vi "Initialize.vi"(8 "error in (no error)":errorcluster, 11 "Bronkhorst Settings in":T1) -> (0 "error out":errorcluster, 2 "No Meter Connected":bool, 3 "Bronkhorst Settings out":T1)   [LabVIEW 2018, in "Bronkhorst M14 Flow Meter.lvlib"]
uses:
  Bronkhorst M14 Flow Meter.lvlib
  Settings Cluster.ctl
  <vilib>/Instr/_visa.llb/VISA Configure Serial Port (Instr).vi
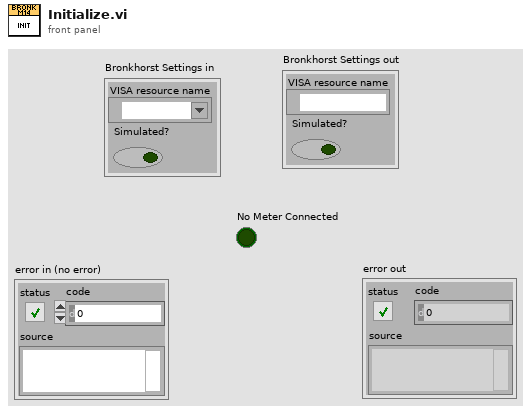
[diagram p1: front panel]
types:
  T1 = typedef "Bronkhorst M14 Flow Meter.lvlib/Settings Cluster.ctl" = cluster{"VISA resource name":refnum<visa-resource-name>, "Simulated?":bool}
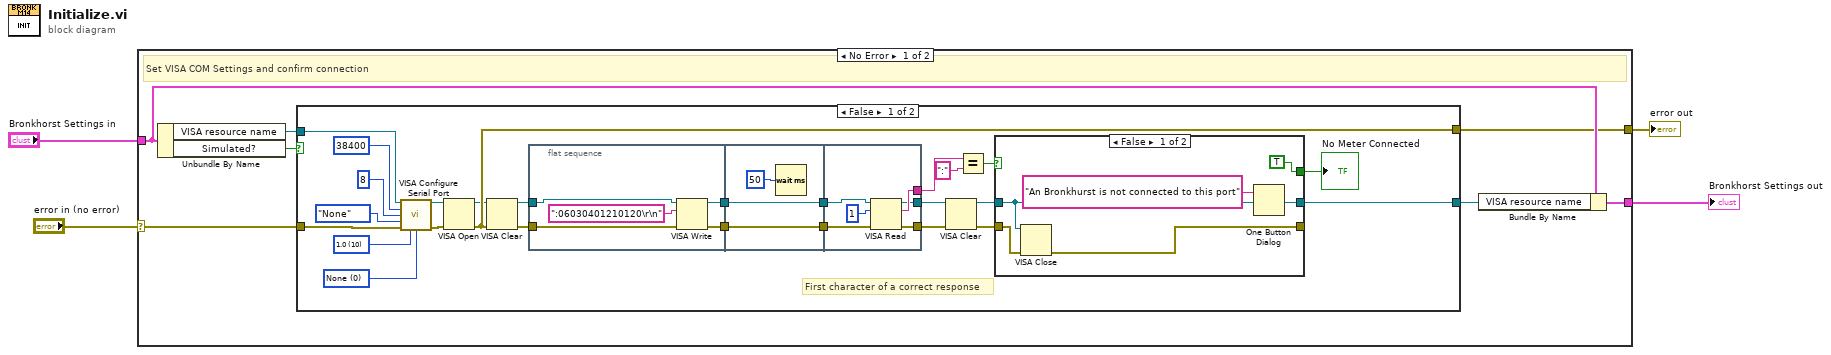
[diagram p0: block diagram]
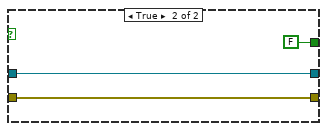
[diagram p2: hidden frame]
diagram:
  n1 = case shown="No Error" "error in (no error)" {
    selector: "error in (no error)" -> [w11 w63]
    tunnel: "Bronkhorst Settings in" -> [w9 w62]
    tunnel: [w5 w63] -> w3
    tunnel: [w8 w62] -> w1
    frame No Error {
      # "Set VISA COM Settings and confirm connection"
      n2 = Unbundle By Name(w9) -> ("VISA resource name"=w7:refnum<visa-resource-name>, "Simulated?"=w10:bool)
      n3 = case shown="False" w10 {
        tunnel: w11 -> [w31 w61]
        tunnel: [w28 w61] -> w5
        tunnel: w7 -> [w29 w60]
        tunnel: [w16 w60] -> w6
        frame False {
          w33 = u16 0 items=["None", "XON/XOFF", "RTS/CTS", "XON/XOFF & RTS/CTS", "DTR/DSR", "XON/XOFF & DTR/DSR"] ("flow control (0:none)")
          w34 = u16 10 items=["1.0"=10, "1.5"=15, "2.0"=20] ("stop bits (10: 1 bit)")
          # "First character of a correct response"
          n4 = call-poly "VISA Configure Serial Port"("VISA resource name"=w29, "baud rate (9600)"=u32 38400, "data bits (8)"=u16 8, "parity (0:none)"=enum16{"None", "Odd", "Even", "Mark", "Space"}."None", "error in (no error)"=w31, "stop bits (10: 1 bit)"=w34, "flow control (0:none)"=w33) -> ("VISA resource name out"=w30:refnum<visa-resource-name>, "error out"=w32:errorcluster)  [unwired: 7 in]
          n5 = VISA Open(error in (no error)=w32, VISA resource name=w30) -> (VISA resource name=w13:refnum<visa-resource-name>, error out=w28:errorcluster)  [unwired: 3 in]
          n6 = VISA Clear(VISA resource name=w13, error in (no error)=w28) -> (VISA resource name out=w14:refnum<visa-resource-name>, error out=w15:errorcluster)
          n7 = flat-sequence {
            tunnel: w15 -> [w42]
            tunnel: [w40] -> w27
            tunnel: [w39] -> w26
            tunnel: w14 -> [w38]
            tunnel: w27 -> [w45]
            tunnel: [w45] -> w25
            tunnel: w26 -> [w44]
            tunnel: [w44] -> w24
            tunnel: [w51] -> w18
            tunnel: [w50] -> w22
            tunnel: [w49] -> w17
            tunnel: w25 -> [w48]
            tunnel: w24 -> [w47]
            frame #0 {
              n8 = VISA Write(VISA resource name=w38, write buffer=":06030401210120\r\n", error in (no error)=w42) -> (VISA resource name out=w40:refnum<visa-resource-name>, error out=w39:errorcluster)  [unwired: 1 out]
            }
            frame #1 {
              n9 = Wait (ms)(milliseconds to wait=u32 50) -> ()  [unwired: 1 out]
            }
            frame #2 {
              n10 = VISA Read(VISA resource name=w48, byte count=u32 1, error in (no error)=w47) -> (VISA resource name out=w49:refnum<visa-resource-name>, read buffer=w50:string, error out=w51:errorcluster)  [unwired: 1 out]
            }
          }
          n11 = VISA Clear(VISA resource name=w17, error in (no error)=w18) -> (VISA resource name out=w19:refnum<visa-resource-name>, error out=w20:errorcluster)
          n12 = Equal?(x=w22, y=":") -> (x = y?=w23:bool)
          n13 = case shown="False" w23 {
            tunnel: w19 -> [w54 w58]
            tunnel: w20 -> [w55 w59]
            tunnel: [w53 w59] -> _
            tunnel: [w54 w58] -> w16
            tunnel: [TRUE FALSE] -> w12
            frame False {
              n14 = VISA Close(VISA resource name=w54, error in (no error)=w55) -> (error out=w53:errorcluster)
              n15 = One Button Dialog(message="An Bronkhurst is not connected to this port") -> ()  [unwired: 1 in, 1 out]
            }
            frame True {
            }
          }
          "No Meter Connected" <- w12
        }
        frame True {
        }
      }
      n16 = Bundle By Name(cluster=w9, "VISA resource name"=w6) -> (w8:T1)
    }
    frame Error {
    }
  }
  "error out" <- w3
  "Bronkhorst Settings out" <- w1
